vi "DLD project .vi"() -> ()   [LabVIEW 2020]
panel:
  out "Fan":bool
  out "Cooler":bool
  out "Ac":bool
  out "Display temp":dbl
  out "?":dbl(knob) scale=-20.0..50.0
  in  "Temperature sensor":dbl(slide) scale=-20.0..50.0
  # "Temperature Sensing Unit"
  # "Display Unit"
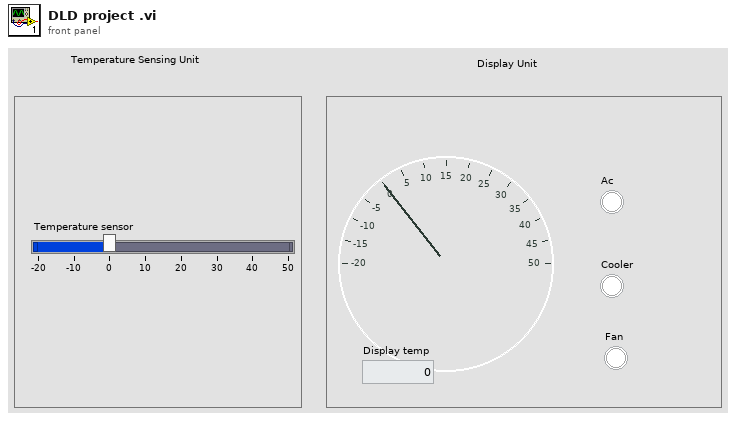
[diagram p1: front panel]
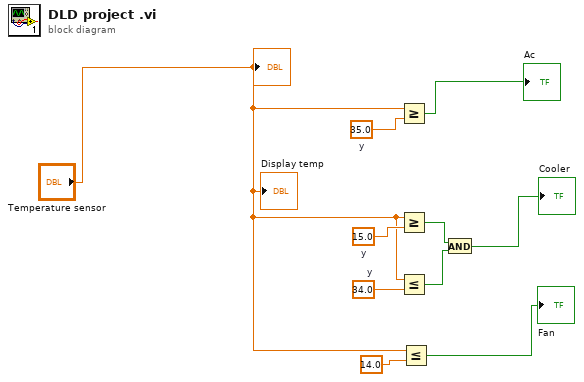
[diagram p0: block diagram]
diagram:
  w7 = 34.0  # y
  w8 = 15.0  # y
  w10 = 35.0  # y
  n1 = Greater Or Equal?(x="Temperature sensor", y=w10) -> (x >= y?=→"Ac":bool)
  n2 = Greater Or Equal?(x="Temperature sensor", y=w8) -> (x >= y?=w6:bool)
  n3 = Less Or Equal?(x="Temperature sensor", y=w7) -> (x <= y?=w5:bool)
  n4 = Less Or Equal?(x="Temperature sensor", y=14.0) -> (x <= y?=→"Fan":bool)
  n5 = And(x=w6, y=w5) -> (x .and. y?=→"Cooler":bool)
  "?" <- "Temperature sensor"
  "Display temp" <- "Temperature sensor"
